vi "Do.vi"(8 "error in (no error)":errorcluster, 10 "Actor in":refnum<class "Actor.lvclass">, 11 "Parse Coords Msg in":refnum<class "Parse Coords Msg.lvclass">) -> (0 "error out":errorcluster, 2 "Actor out":refnum<class "Actor.lvclass">)   [LabVIEW 2018, in "Stage Actor.lvlib" / "Parse Coords Msg.lvclass"]
uses:
  Parse Coords Msg.lvclass
  <vilib>/ActorFramework/Actor/Actor.lvclass
  Stage/Stage.lvclass
  C:/Program Files/National Instruments/LabVIEW 2018/vi.lib/ActorFramework/Actor/Actor.lvclass
  Parse Coords Msg.lvclass/Parse Coords Msg.ctl
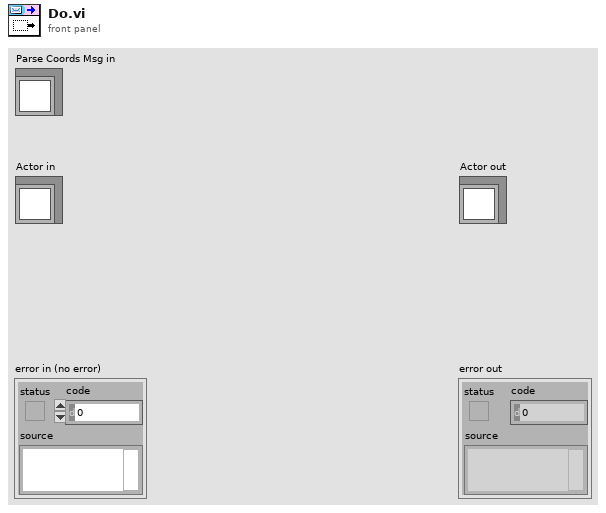
[diagram p1: front panel]
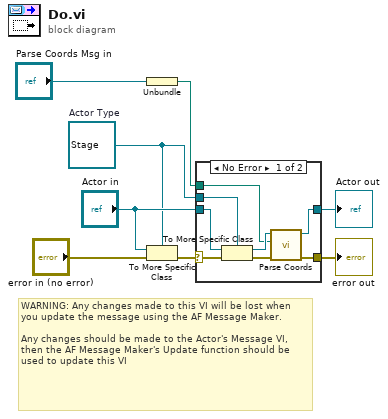
[diagram p0: block diagram]
diagram:
  w3 = refnum<class "Stage.lvclass"> refnum  # Actor Type
  # "WARNING: Any changes made to this VI will be lost when you update the message using the AF Message Maker.\n\nAny changes should be made to the Actor's Message VI, then the AF Message Maker's Update function should be used to update this VI"
  n1 = Unbundle("Parse Coords Msg in") -> (w2:path)
  n2 = To More Specific Class(target class=w3, reference="Actor in", error in="error in (no error)") -> (error out=w7:errorcluster)  [unwired: 1 out]
  n3 = case shown="No Error" w7 {
    selector: w7 -> [w16 w18]
    tunnel: [w11 w18] -> w6
    tunnel: [w10 w17] -> w5
    tunnel: "Actor in" -> [w15 w17]
    tunnel: w3 -> [w14 _]
    tunnel: w2 -> [w9 _]
    frame No Error {
      n4 = To More Specific Class ("Actor Cast")(target class=w14, reference=w15, error in=w16) -> (specific class reference=w13:refnum<class "Stage.lvclass">, error out=w12:errorcluster)
      n5 = call "Parse Coords.vi"("error in (no error)"=w12, "Read Coordinates"=w9, "Stage Actor.lvlib:Stage.lvclass"=w13) -> ("error out"=w11:errorcluster, "Stage Actor.lvlib:Stage.lvclass"=w10:refnum<class "Stage.lvclass">)  [unwired: 7 in]
    }
    frame Error {
    }
  }
  "error out" <- w6
  "Actor out" <- w5
